vi "Waveform_Replace Waveform.vi"(8 "Error":errorcluster, 9 "Waveform to replace":T1, 11 "Waveform":T1) -> (0 "Error Out":errorcluster, 3 "Waveform Out":T1)   [LabVIEW 2020]
doc: "Retrieves a subset of a waveform at a specified time or index. You must manually select the polymorphic instance you want to use."
uses:
  Universal Controls/Waveform_Data.ctl
  <vilib>/Waveform/WDTOps.llb/WDT Get Final Time Value DBL.vi
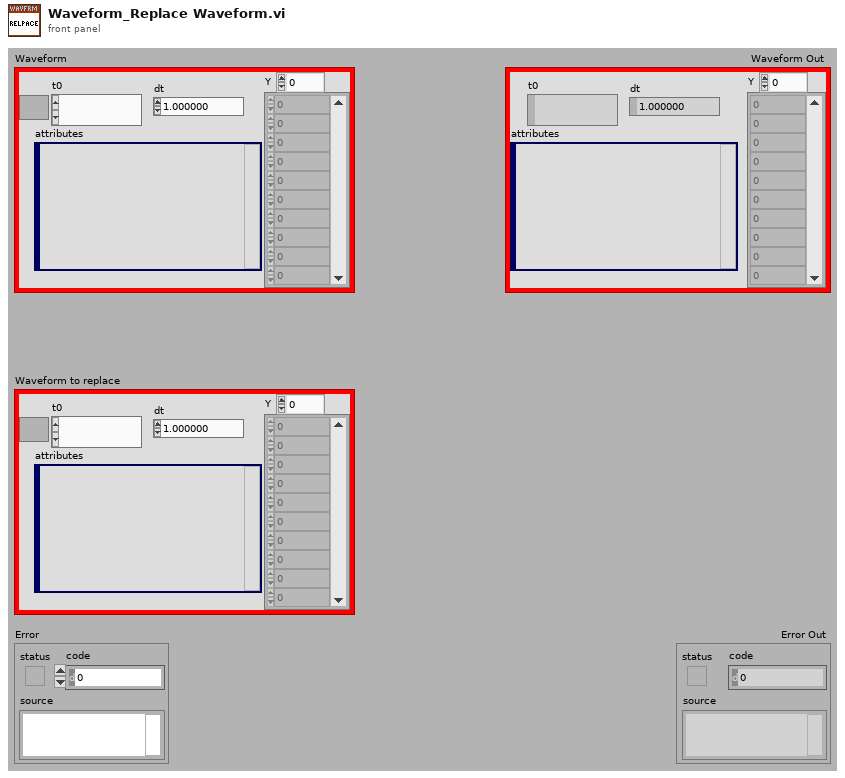
[diagram p1: front panel]
types:
  T1 = typedef "Waveform_Data.ctl" = waveform(dbl)
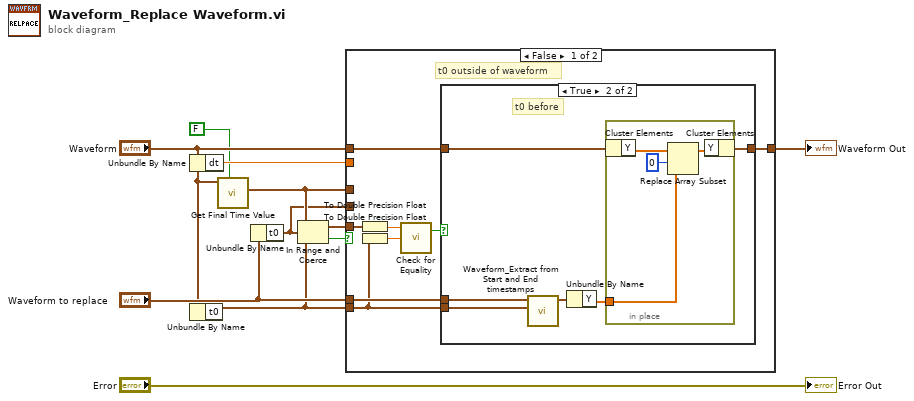
[diagram p0: block diagram]
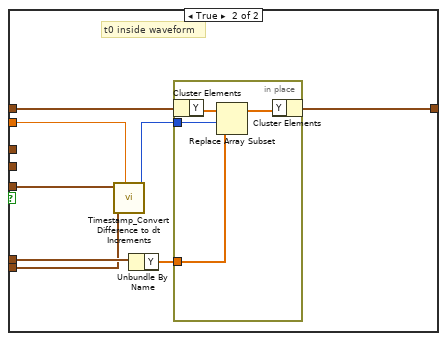
[diagram p3: hidden frame]
diagram:
  n1 = Unbundle By Name("Waveform") -> ("dt"=w9:dbl)
  n2 = Unbundle By Name("Waveform") -> ("t0"=w6:timestamp)
  n3 = call-poly <vilib>:"Get Final Time Value.vi"("open interval? (T)"=FALSE, "waveform in"="Waveform") -> ("tf"=w4:timestamp)  [unwired: 7 in, 2 out]
  n4 = Unbundle By Name("Waveform to replace") -> ("t0"=w3:timestamp)
  n5 = In Range and Coerce(upper limit=w4, x=w3, lower limit=w6) -> (coerced(x)=w7:timestamp, In Range?=w11:bool)
  n6 = case shown="False" w11 {
    tunnel: "Waveform" -> [w19 w37]
    tunnel: "Waveform to replace" -> [w17 w34]
    tunnel: w9 -> [_ w38]
    tunnel: [w18 w33] -> w8
    tunnel: w7 -> [w16 w31]
    tunnel: w6 -> [w15 w32]
    tunnel: w4 -> [_ _]
    tunnel: w3 -> [_ _]
    frame False {
      # "t0 outside of waveform"
      n7 = To Double Precision Float(number=w16) -> (double precision float=w13:dbl)
      n8 = To Double Precision Float(number=w15) -> (double precision float=w14:dbl)
      n9 = call <vilib>:"Check for Equality.vi"("n2"=w14, "n1"=w13) -> ("equal?"=w12:bool)  [unwired: 1 in, 1 out]
      n10 = case shown="True" w12 {
        tunnel: w19 -> [w20 w24]
        tunnel: [w20 w23] -> w18
        tunnel: w17 -> [_ w26]
        tunnel: w15 -> [_ w25]
        frame False {
          # "t0 past tf"
        }
        frame True {
          # "t0 before"
          n11 = call "Waveform_Extract from Start and End timestamps.vi"("T0 Time"=w25, "Waveform"=w26) -> ("Waveform Out"=w22:T1)  [unwired: 6 in, 3 out]
          n12 = Unbundle By Name(w22) -> ("Y"=w21:dbl[])
          n13 = in-place {
            in-place-border: w21 -> [w28]
            n14 = in-place-cluster #1(w24) -> ("Y"=w30:dbl[])
            n15 = Replace Array Subset(array=w30, new element=w28, index=0) -> (w29:dbl[])
            n16 = in-place-cluster #1("Y"=w29) -> (w23:T1)
          }
        }
      }
    }
    frame True {
      # "t0 inside waveform"
      n17 = call "Timestamp_Convert Difference to dt Increments.vi"("Dt"=w38, "Start Time"=w32, "End Time"=w31) -> ("Nearest Dt Increment Out"=w35:i32)  [unwired: 6 in, 2 out]
      n18 = Unbundle By Name(w34) -> ("Y"=w36:dbl[])
      n19 = in-place {
        in-place-border: w36 -> [w39]
        in-place-border: w35 -> [w40]
        n20 = in-place-cluster #2(w37) -> ("Y"=w42:dbl[])
        n21 = Replace Array Subset(array=w42, new element=w39, index=w40) -> (w41:dbl[])
        n22 = in-place-cluster #2("Y"=w41) -> (w33:T1)
      }
    }
  }
  "Waveform Out" <- w8
  "Error Out" <- "Error"
